vi "SelectProject.vi"() -> (2 "OK？":bool, 3 "ProjectName":string)   [LabVIEW 2018, in "TestStand Simple UI.lvlib"]
uses:
  TestExec.llb/TestStand Simple UI.lvlib
panel:
  in  "String":string
  in  "Cancel Button":bool
  in  "OK Button":bool
  in  "项目文件":i32(listbox)
  in  "项目名称/代号":i32(listbox)
  # "选择测试项目"
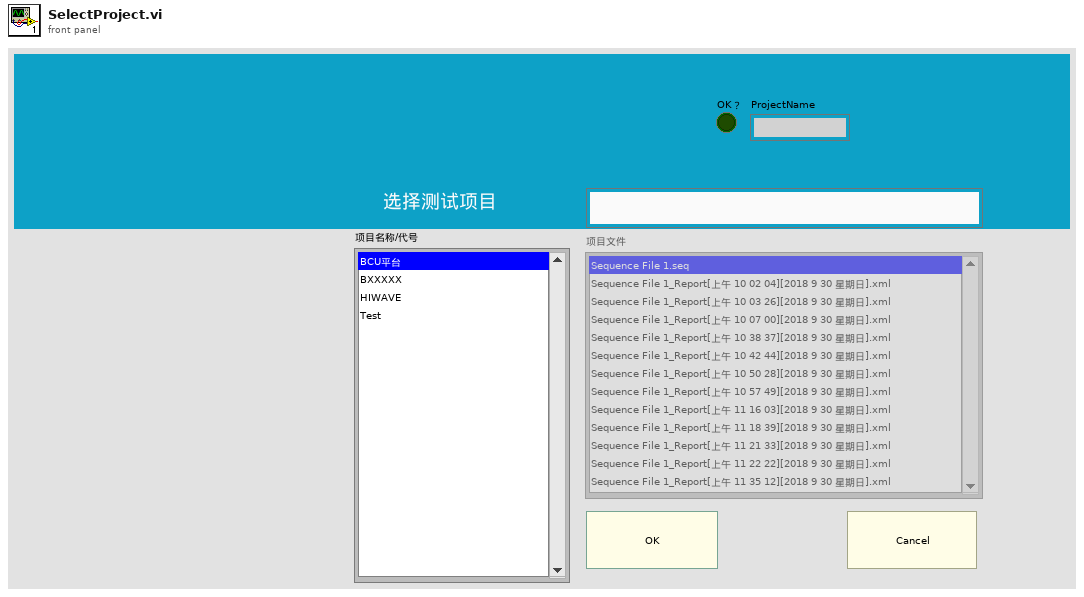
[diagram p1: front panel]
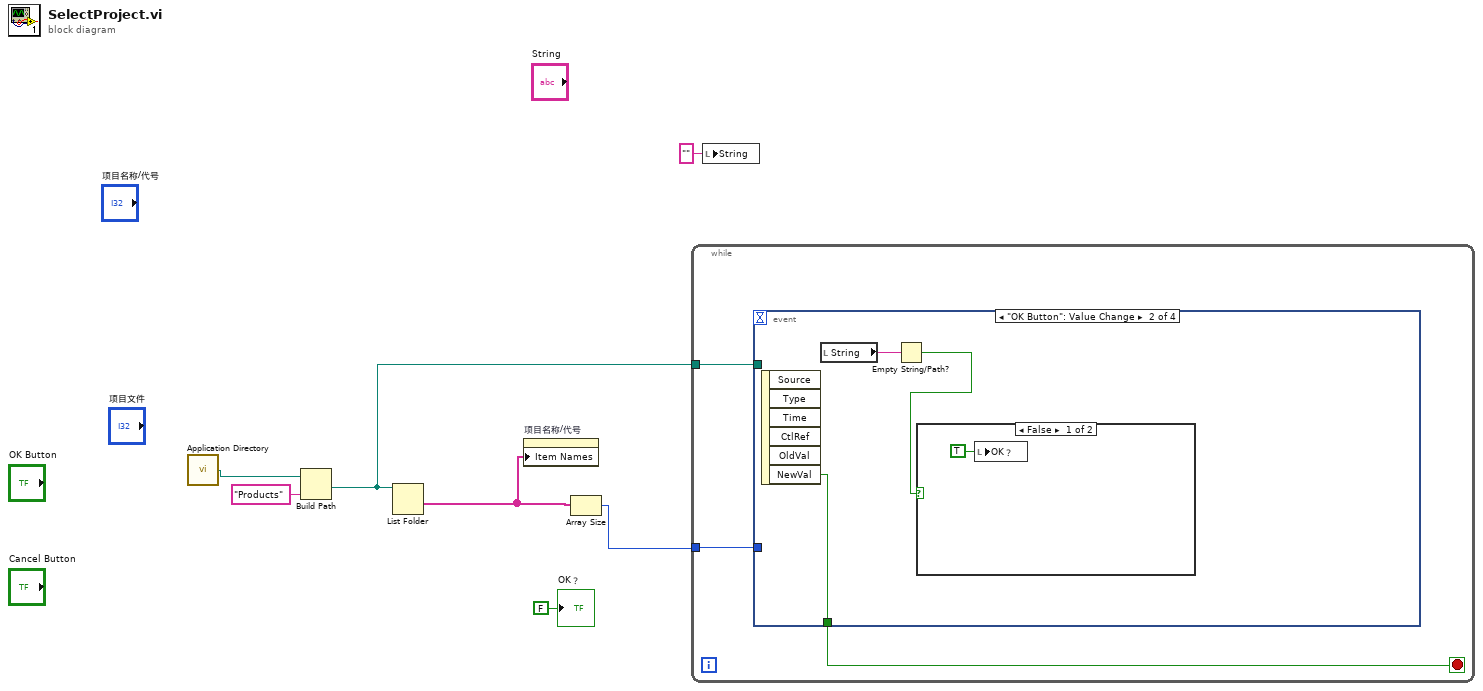
[diagram p0: block diagram]
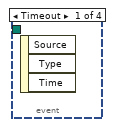
[diagram p2: hidden frame]
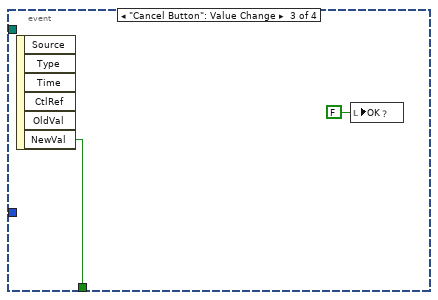
[diagram p4: hidden frame]
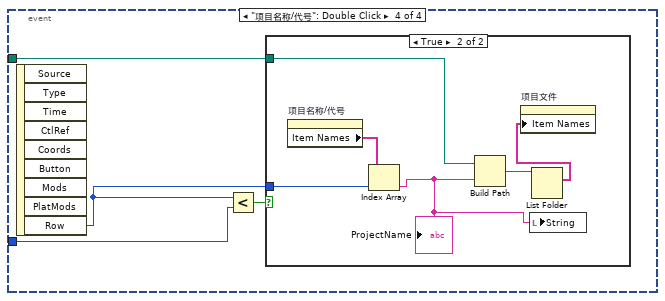
[diagram p5: hidden frame]
diagram:
  n1 = call <vilib>:"Application Directory.vi"() -> ("Application Directory"=w7:path)
  n2 = Build Path(base path=w7, name or relative path="Products" ("名称或相对路径")) -> (appended path=w3:path)
  n3 = List Folder(path=w3) -> (folder names=w5:string[])  [unwired: 3 in, 3 out]
  n4 = property on="项目名称/代号" class="LstBox (strict)"("Item Names"=w5) -> ()  [unwired: 2 in, 2 out]
  n5 = Array Size(array=w5) -> (size(s)=w4:i32)
  n6 = while {
    tunnel: w4 -> [w9]
    tunnel: w3 -> [w8]
    stop <- w10 stop-if-true
    n7 = event shown="[1] \"OK Button\": Value Change" {
      selector: _ -> [_ _ _ _]
      dyn-events: _ -> [_ _ _ _]
      timeout: _ -> [_ _ _ _]
      tunnel: [_ w13 w16 _] -> w10
      tunnel: w9 -> [_ _ _ w20]
      tunnel: w8 -> [_ _ _ w17]
      event Timeout {
        n8 = event-data() -> ()  [unwired: 1 in, 3 out]
      }
      event "OK Button": Value Change {
        n9 = event-data() -> ("NewVal"=w13:bool)  [unwired: 1 in, 5 out]
        n10 = local read "String"() -> (w12:string)
        n11 = Empty String/Path?(string/path=w12) -> (empty?=w11:bool)
        n12 = case shown="False" w11 {
          frame False {
            n13 = local write "OK？"(TRUE ("OK？")) -> ()
          }
          frame True {
          }
        }
      }
      event "Cancel Button": Value Change {
        n14 = event-data() -> ("NewVal"=w16:bool)  [unwired: 1 in, 5 out]
        n15 = local write "OK？"(FALSE ("OK？")) -> ()
      }
      event "项目名称/代号": Double Click {
        n16 = event-data() -> ("Row"=w18:i32)  [unwired: 1 in, 8 out]
        n17 = Less?(x=w18, y=w20) -> (x < y?=w19:bool)
        n18 = case shown="True" w19 {
          tunnel: w18 -> [_ w25]
          tunnel: w17 -> [_ w24]
          frame False {
          }
          frame True {
            n19 = property on="项目名称/代号" class="LstBox (strict)"() -> ("Item Names"=w26:string[])  [unwired: 2 in, 2 out]
            n20 = Index Array(array=w26, index=w25) -> (element=w21:string)
            "ProjectName" <- w21
            n21 = Build Path(base path=w24, name or relative path=w21) -> (appended path=w23:path)
            n22 = local write "String"(w21) -> ()
            n23 = List Folder(path=w23) -> (filenames=w22:string[])  [unwired: 3 in, 3 out]
            n24 = property on="项目文件" class="LstBox (strict)"("Item Names"=w22) -> ()  [unwired: 2 in, 2 out]
          }
        }
      }
    }
  }
  n25 = local write "String"("" ("String")) -> ()
  "OK？" <- FALSE ("OK？")
